vi "Color Threshold.vi"() -> ()   [LabVIEW 2014]
doc: "This example shows the advantages of using the HSL color space over the RGB color space to perform color inspection in certain situations."
uses:
  <vilib>/vision/NI_Vision_Development_Module.lvlib
panel:
  in  "Stop":bool
  in  "Test Image":enum32{"Image 1", "Image 2"}(radio)
  in  "Threshold Color Mode":enum32{"RGB", "HSL"}(radio)=enum."HSL"
  in  "Blue or Luminance":cluster{i32, i32}(slide)={20, 217} scale=0.0..255.0
  in  "Green or Saturation":cluster{i32, i32}(slide)={20, 233} scale=0.0..255.0
  in  "Red or Hue":cluster{i32, i32}(slide)={42, 99} scale=0.0..255.0
  out "Original Image":T1(plugin-control)
  out "Threshold Image":T1(plugin-control)
  # "Overview: Demonstrates how to use the IMAQ Color Threshold function to produce a binary image from a color image.\nRequirements: Vision Development Software.\nInstructions:\n1. Run the VI and change the Test Image to use different images with the same threshold ranges.\n2. Adjust the sliders to change the threshold ranges. Notice that HSL is a better Threshold Color Mode to find specific colors with lighting variations."
  # "Minimum"
  # "Maximum"
  # "Minimum"
  # "Maximum"
  # "Minimum"
  # "Maximum"
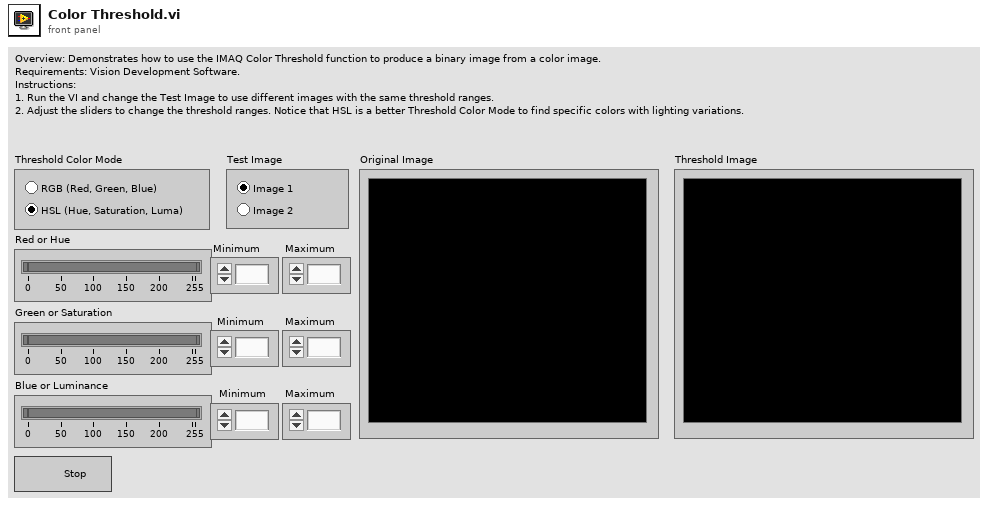
[diagram p1: front panel]
types:
  T1 = typedef "IMAQ Image.ctl" = refnum<image>
  T2 = typedef "Image Type" = u32
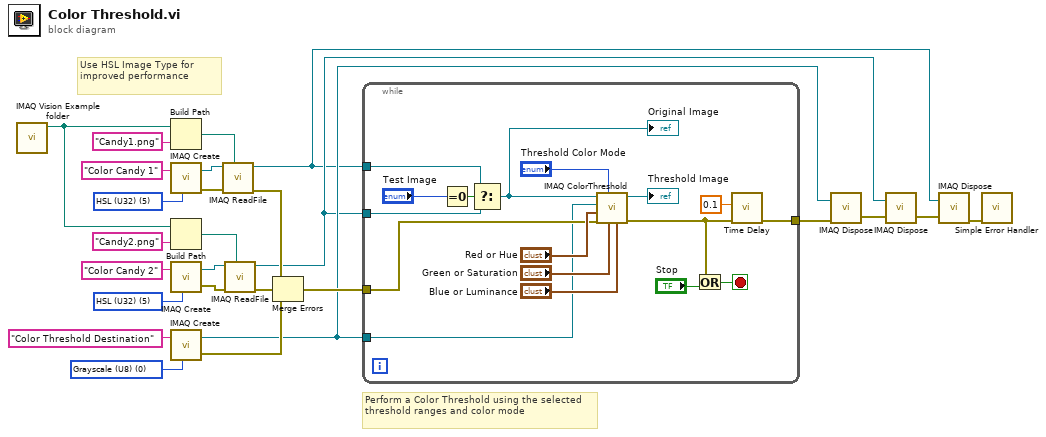
[diagram p0: block diagram]
diagram:
  w4 = T2 5 items=["Grayscale (U8)", "Grayscale (I16)", "Grayscale (SGL)", "Complex (CSG)", "RGB (U32)", "HSL (U32)", "RGB (U64)", "Grayscale (U16)"] ("Image Type")
  w6 = T2 0 items=["Grayscale (U8)", "Grayscale (I16)", "Grayscale (SGL)", "Complex (CSG)", "RGB (U32)", "HSL (U32)", "RGB (U64)", "Grayscale (U16)"] ("Image Type")
  w7 = T2 5 items=["Grayscale (U8)", "Grayscale (I16)", "Grayscale (SGL)", "Complex (CSG)", "RGB (U32)", "HSL (U32)", "RGB (U64)", "Grayscale (U16)"] ("Image Type")
  # "Use HSL Image Type for improved performance"
  # "Perform a Color Threshold using the selected threshold ranges and color mode"
  n1 = call "IMAQ Vision Example folder.vi"() -> ("Example Image Path"=w5:path)  [unwired: 11 in]
  n2 = Build Path(base path=w5, name or relative path="Candy1.png") -> (appended path=w22:path)
  n3 = call "IMAQ Create"("Image Name"="Color Candy 1", "Image Type"=w4) -> ("New Image"=w21:T1, "error out"=w20:errorcluster)  [unwired: 3 in]
  n4 = Build Path(base path=w5, name or relative path="Candy2.png") -> (appended path=w16:path)
  n5 = call "IMAQ Create"("Image Name"="Color Candy 2", "Image Type"=w7) -> ("New Image"=w19:T1, "error out"=w18:errorcluster)  [unwired: 3 in]
  n6 = call "IMAQ Create"("Image Name"="Color Threshold Destination", "Image Type"=w6) -> ("New Image"=w3:T1, "error out"=w12:errorcluster)  [unwired: 3 in]
  n7 = call "IMAQ ReadFile"("File Path"=w22, "error in (no error)"=w20, "Image"=w21) -> ("error out"=w13:errorcluster, "Image Out"=w1:T1)  [unwired: 4 in, 3 out]
  n8 = call "IMAQ ReadFile"("File Path"=w16, "error in (no error)"=w18, "Image"=w19) -> ("error out"=w14:errorcluster, "Image Out"=w2:T1)  [unwired: 4 in, 3 out]
  n9 = Merge Errors(w13, w14, w12) -> (w11:errorcluster)
  n10 = while {
    tunnel: w3 -> [w27]
    tunnel: w1 -> [w39]
    tunnel: w2 -> [w38]
    tunnel: [w29] -> w15
    tunnel: w11 -> [w30]
    stop <- w35 stop-if-true
    n11 = Equal To 0?(x="Test Image") -> (x = 0?=w40:bool)
    n12 = Select(t=w39, s=w40, f=w38) -> (s? t:f=w34:T1)
    "Original Image" <- w34
    n13 = call "IMAQ ColorThreshold"("Blue or Luma or Val or Inten Range"="Blue or Luminance", "Green or Sat Range"="Green or Saturation", "Color Mode"="Threshold Color Mode", "error in (no error)"=w30, "Red or Hue Range"="Red or Hue", "Image Dst"=w27, "Image Src"=w34) -> ("error out"=w32:errorcluster, "Image Dst Out"=→"Threshold Image":T1)  [unwired: 3 in]
    n14 = Or(x=w32, y="Stop") -> (x .or. y?=w35:bool)
    n15 = call "Time Delay"("error in (no error)"=w32, "Delay Time (s)"=0.1) -> ("error out"=w29:errorcluster)  [unwired: 9 in]
  }
  n16 = call "IMAQ Dispose"("Image"=w3, "error in (no error)"=w15) -> ("error out"=w10:errorcluster)  [unwired: 4 in]
  n17 = call "IMAQ Dispose"("Image"=w2, "error in (no error)"=w10) -> ("error out"=w9:errorcluster)  [unwired: 4 in]
  n18 = call "IMAQ Dispose"("Image"=w1, "error in (no error)"=w9) -> ("error out"=w8:errorcluster)  [unwired: 4 in]
  n19 = call <vilib>:"Simple Error Handler.vi"("error in (no error)"=w8) -> ()  [unwired: 4 in, 5 out]
